vi "roverView.vi"() -> ()   [LabVIEW 2020]
uses:
  globalVariables.vi
panel:
  in  "Simulation stop":bool
  out "Back right wheel":dbl(graph)
  out "Back left wheel":dbl(graph)
  out "Front right wheel":dbl(graph)
  out "Front left wheel":dbl(graph)
  out "Velocity of the rover's left-side wheels":dbl(graph)
  out "Rover wheel velocity on the right side":string
  out "Scientific notation":dbl
  out "Scientific notation":dbl
  out "Rover wheel velocity on the left side":string
  out "Velocity of the rover's right-side wheels":dbl(graph)
  out "standard output 2":string
  out "ASCII Char 3":i16
  out "Character 2":string
  out "System user":string
  out "Simulation time":dbl
  out "Movement log":string
  out "Keys pressed log":string
  out "Key pressed":string
  out "Detected movement indicator":string
  out "ASCII Char 2":i16
  out "ASCII Char":i16
  out "Character":string
  out "standard output":string
  # "Rover control"
  # "Logs"
  # "Wheel movement charts"
  # "Movement data"
  # "Velocity charts"
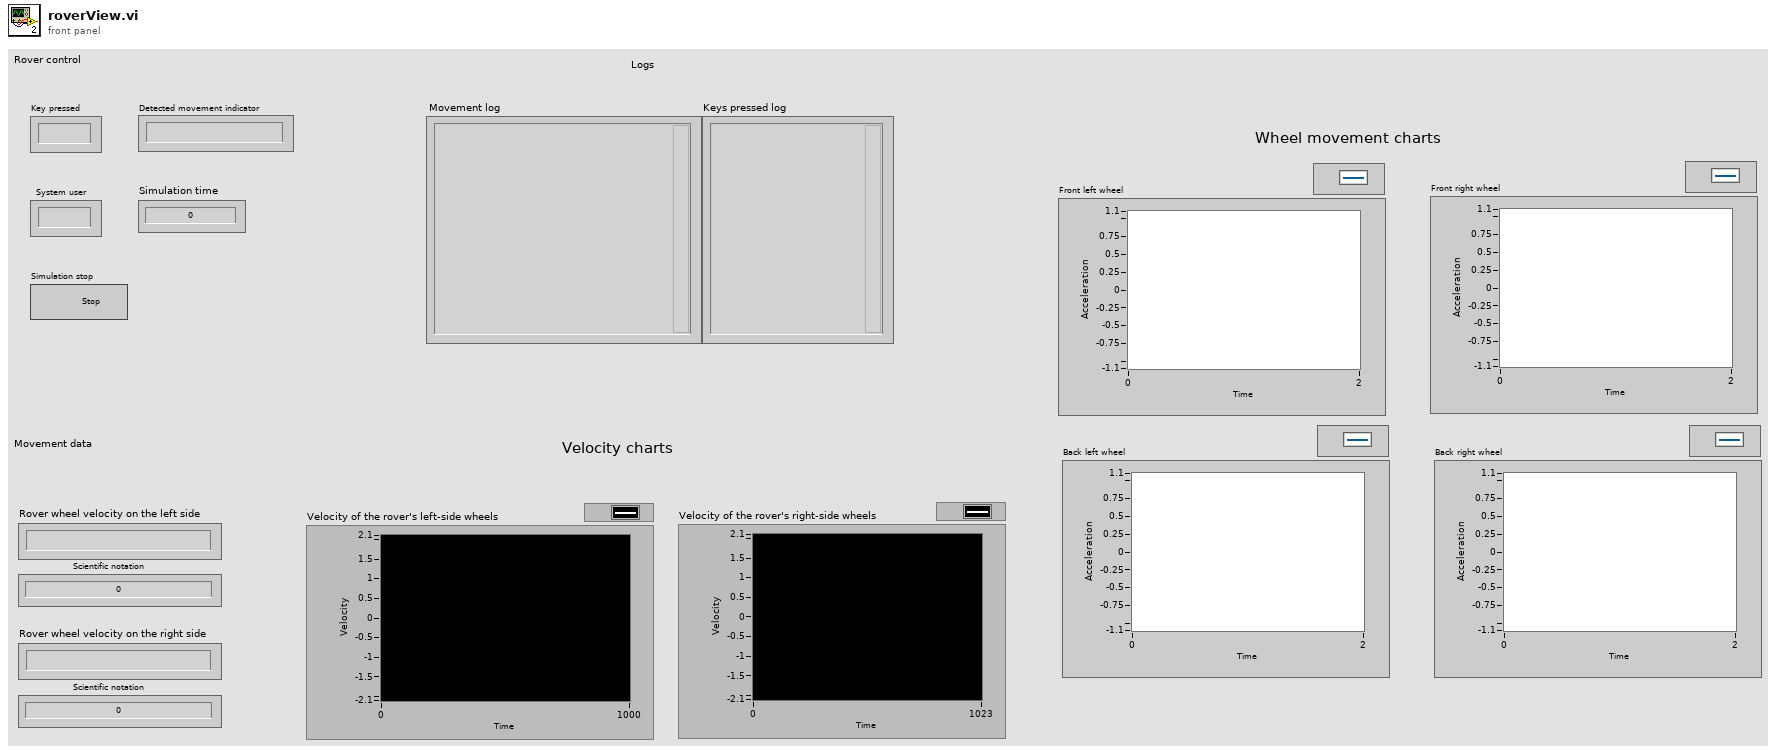
[diagram p1: front panel]
types:
  T1 = enum16{"Start", "Process 1", "Process 2", "Stop"}
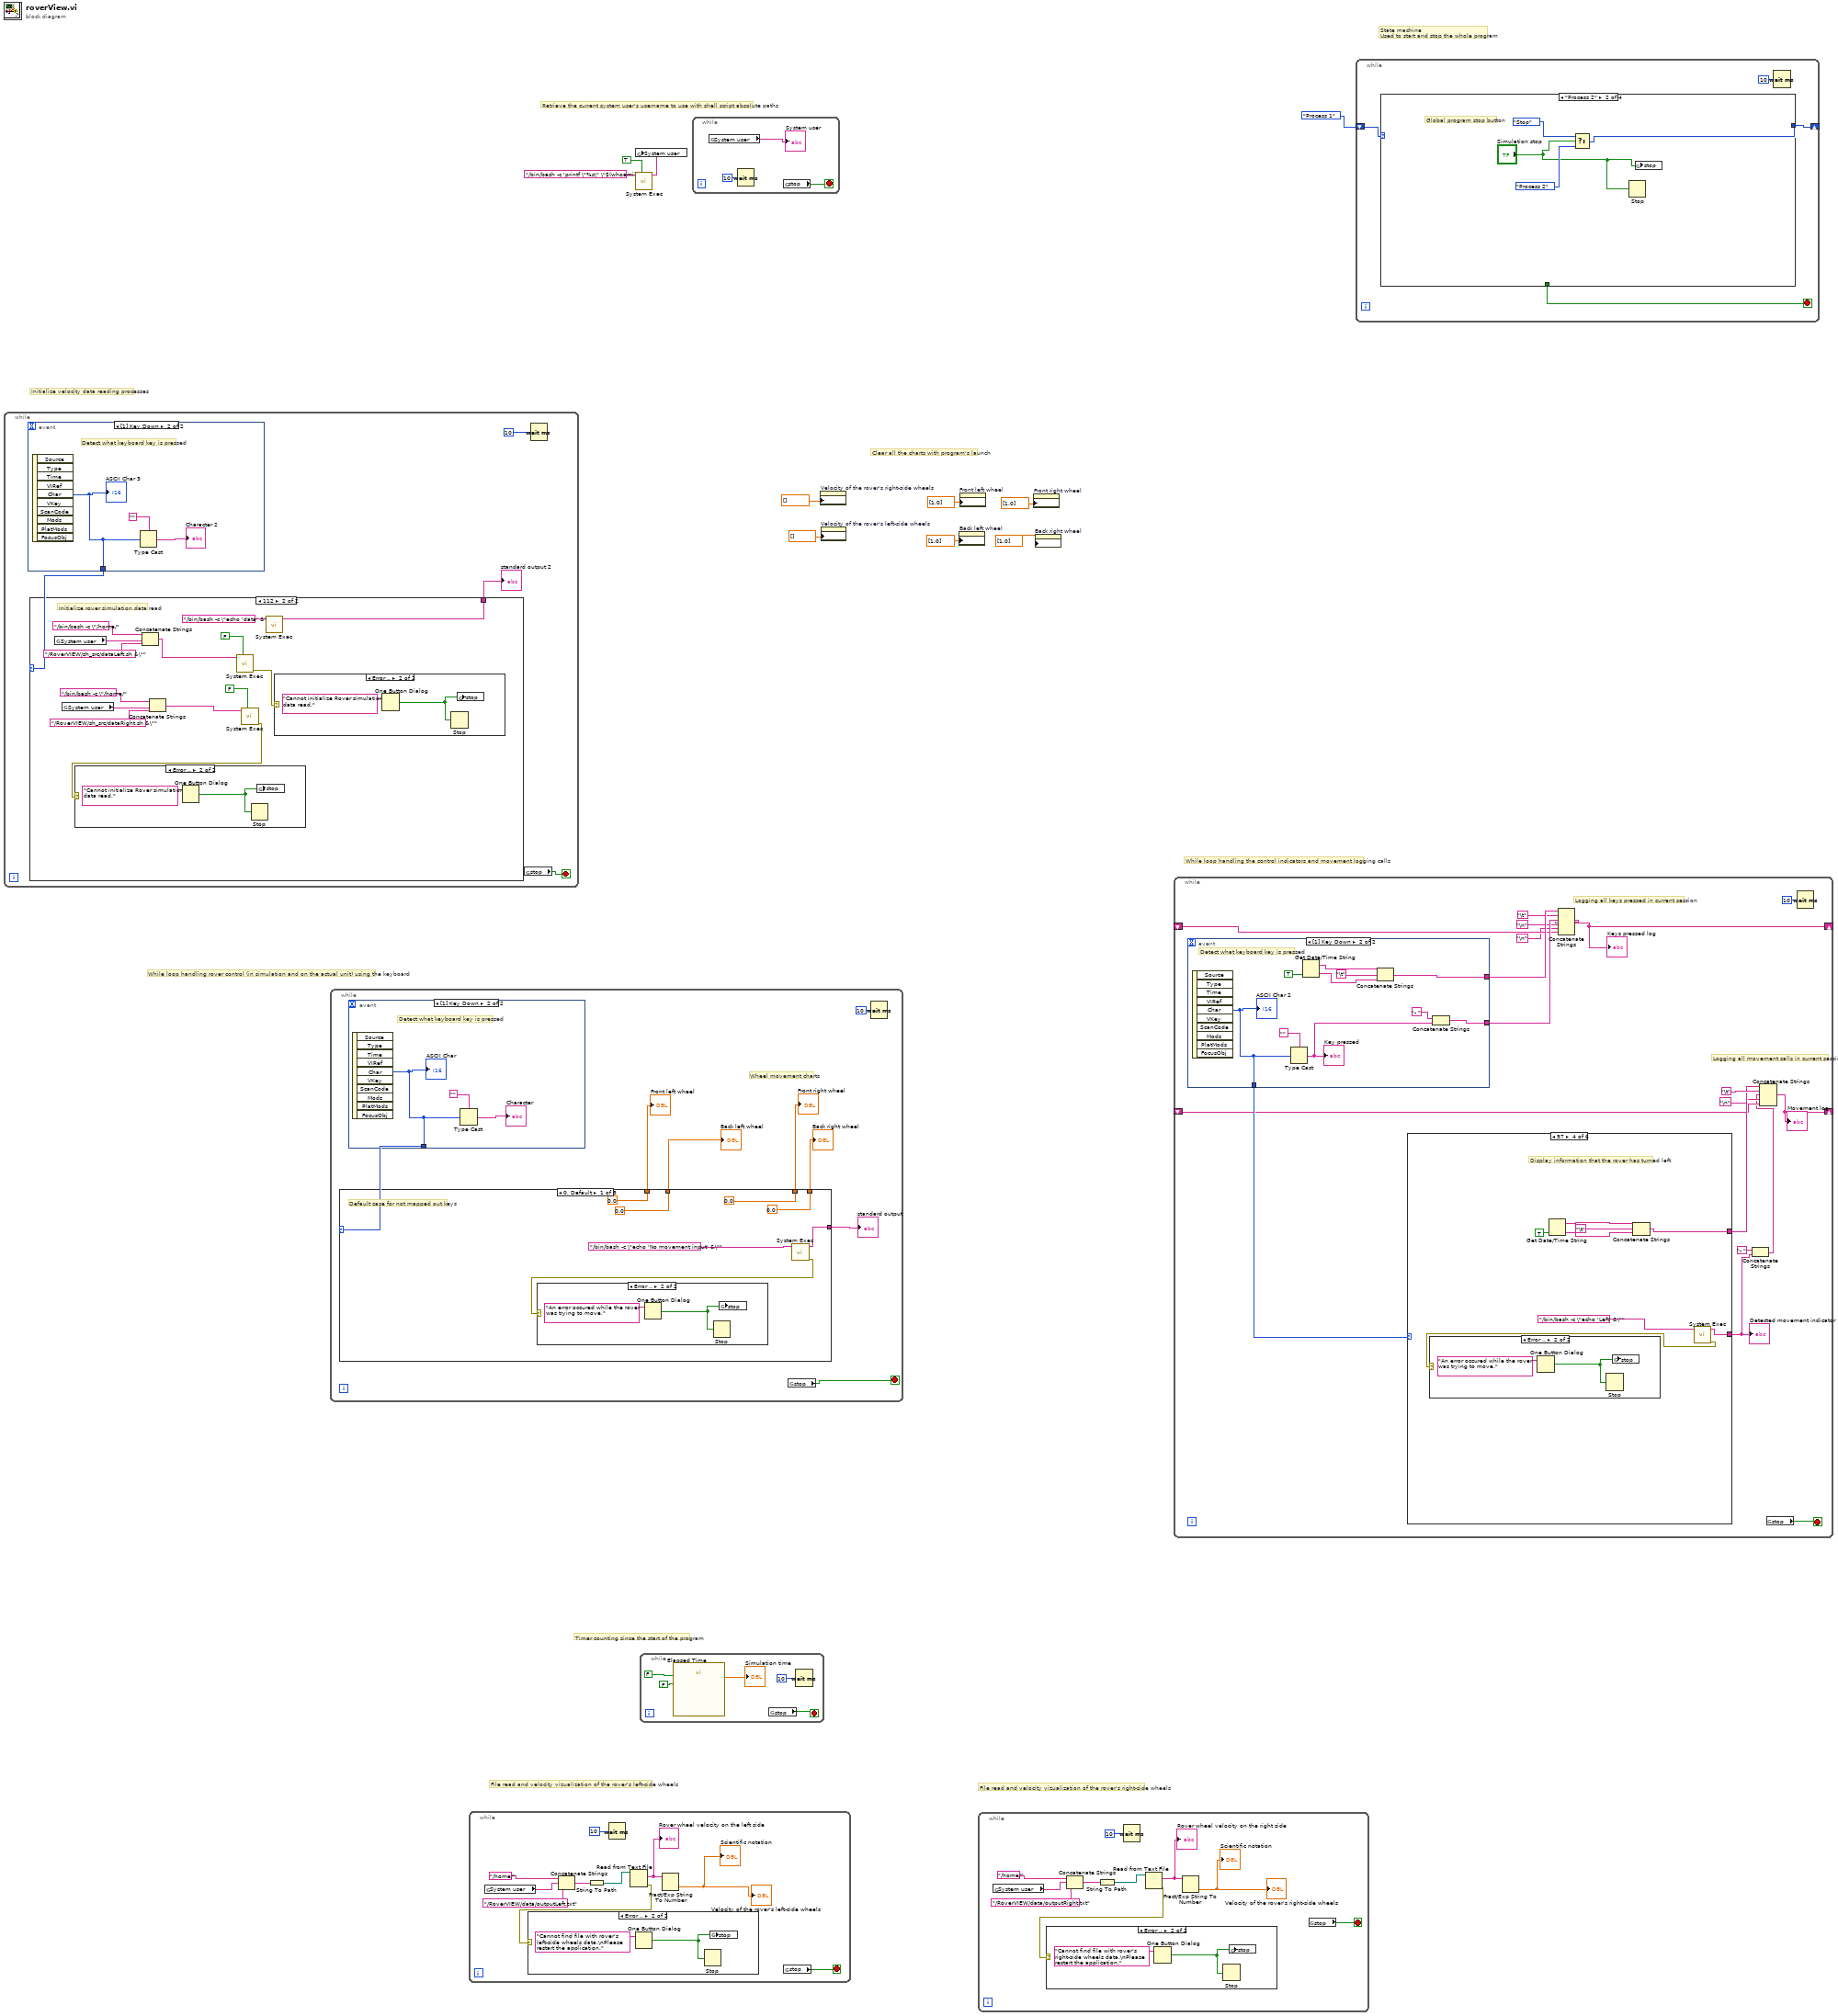
[diagram p0: block diagram]
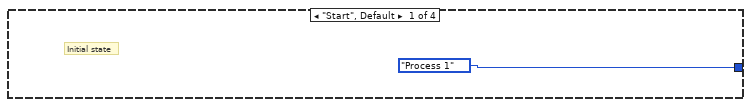
[diagram p2: hidden frame]
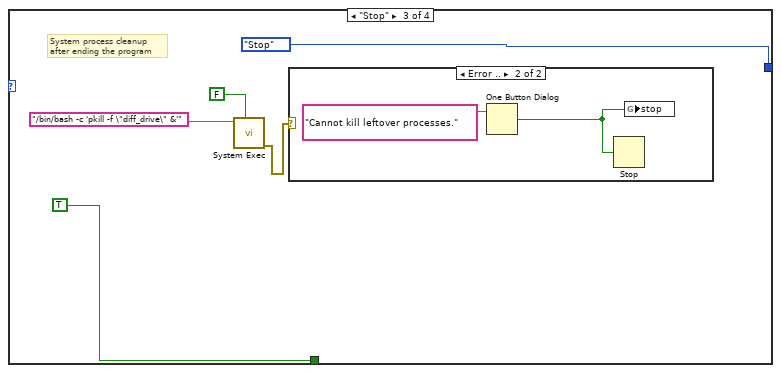
[diagram p3: hidden frame]
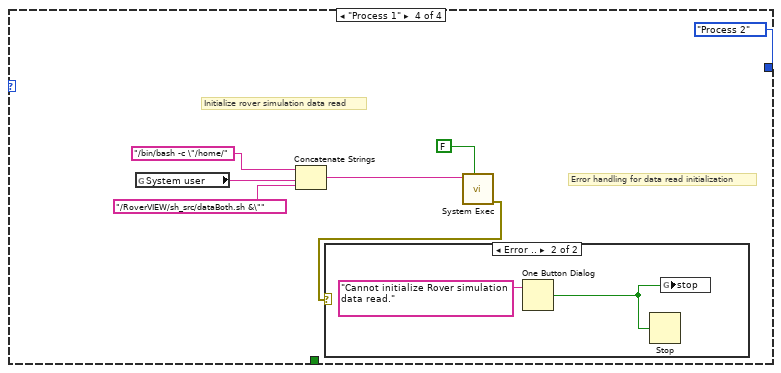
[diagram p5: hidden frame]
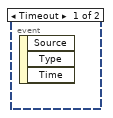
[diagram p7: hidden frame]
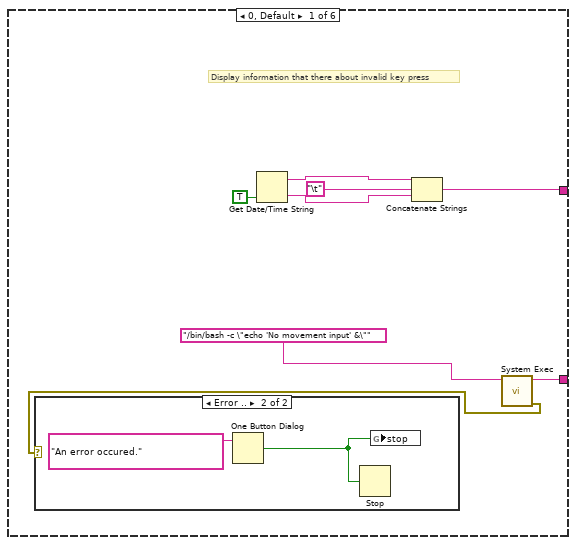
[diagram p13: hidden frame]
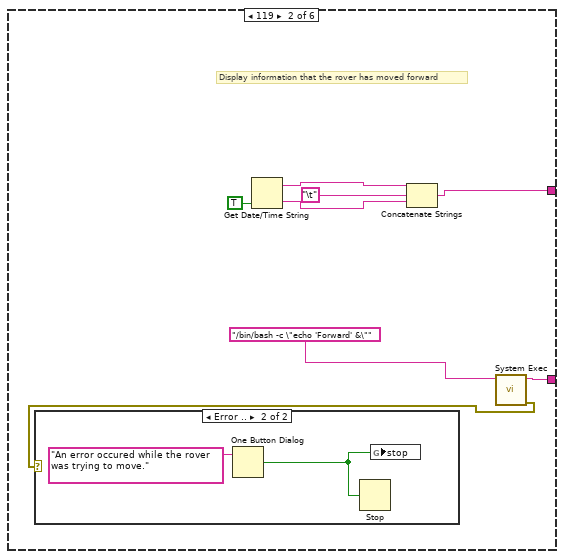
[diagram p15: hidden frame]
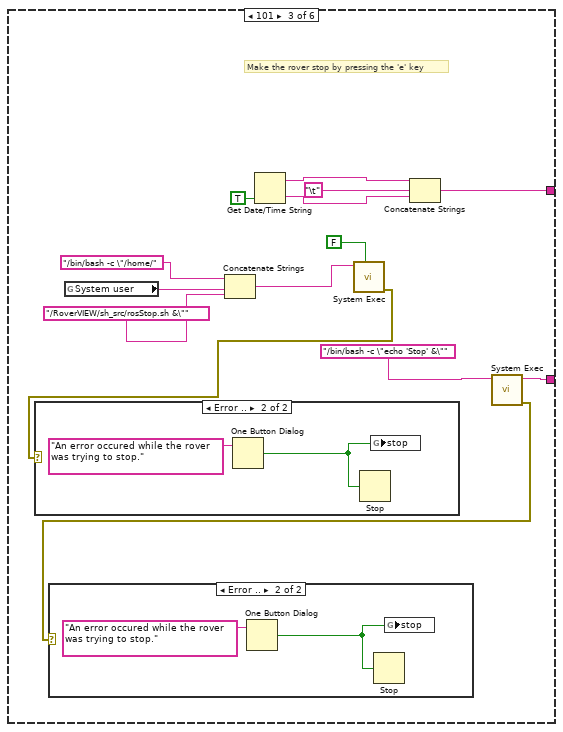
[diagram p17: hidden frame]
diagram:
  # "State machine\nUsed to start and stop the whole program"
  # "Clear all the charts with program's launch"
  # "Initialize velocity data reading processes"
  # "File read and velocity vizualization of the rover's right-side wheels"
  # "File read and velocity vizualization of the rover's left-side wheels"
  # "Timer counting since the start of the program"
  # "Retrieve the current system user's username to use with shell script absolute paths"
  # "While loop handling the control indicators and movement logging calls"
  # "While loop handling rover control (in simulation and on the actual unit) using the keyboard"
  n1 = while {
    stop <- w11 stop-if-true
    n2 = event shown="[1] Key Down" {
      selector: _ -> [_ _]
      dyn-events: _ -> [_ _]
      timeout: _ -> [_ _]
      tunnel: [_ w15] -> w14
      event Timeout {
        n3 = event-data() -> ()  [unwired: 1 in, 3 out]
      }
      event Key Down {
        # "Detect what keyboard key is pressed"
        n4 = event-data() -> ("Char"=w15:i16)  [unwired: 1 in, 9 out]
        "ASCII Char 3" <- w15
        n5 = Type Cast(type="", x=w15) -> (*(type *) &x=→"Character 2":string)
      }
    }
    n6 = case shown="112" w14 {
      tunnel: [_ w28] -> w13
      frame 0, Default {
        # "Initial state"
      }
      frame 112 {
        # "Initialize rover simulation data read"
        n7 = global read "globalVariables.vi" "System user"() -> (w22:string)
        n8 = global read "globalVariables.vi" "System user"() -> (w26:string)
        n9 = Concatenate Strings("/bin/bash -c \"/home/", w22, "/RoverVIEW/sh_src/dataLeft.sh &\"") -> (w20:string)
        n10 = Concatenate Strings("/bin/bash -c \"/home/", w26, "/RoverVIEW/sh_src/dataRight.sh &\"") -> (w24:string)
        n11 = call <vilib>:"System Exec.vi"("wait until completion? (T)"=FALSE, "command line"=w20) -> ("error out"=w18:errorcluster)  [unwired: 6 in, 3 out]
        n12 = call <vilib>:"System Exec.vi"("wait until completion? (T)"=FALSE, "command line"=w24) -> ("error out"=w19:errorcluster)  [unwired: 6 in, 3 out]
        n13 = case shown="Error .." w19 {
          frame No Error {
          }
          frame Error {
            n14 = One Button Dialog(message="Cannot initialize Rover simulation data read.") -> (true=w34:bool)  [unwired: 1 in]
            n15 = Stop(stop? (T)=w34) -> ()
            n16 = global write "globalVariables.vi" "stop"(w34) -> ()
          }
        }
        n17 = call <vilib>:"System Exec.vi"("command line"="/bin/bash -c \"echo 'data' &\"") -> ("standard output"=w28:string)  [unwired: 7 in, 3 out]
        n18 = case shown="Error .." w18 {
          frame No Error {
          }
          frame Error {
            n19 = One Button Dialog(message="Cannot initialize Rover simulation data read.") -> (true=w32:bool)  [unwired: 1 in]
            n20 = Stop(stop? (T)=w32) -> ()
            n21 = global write "globalVariables.vi" "stop"(w32) -> ()
          }
        }
      }
    }
    "standard output 2" <- w13
    n22 = global read "globalVariables.vi" "stop"() -> (w11:bool)
    n23 = Wait (ms)(milliseconds to wait=u32 10) -> ()  [unwired: 1 out]
  }
  n24 = while {
    stop <- w36 stop-if-true
    # "Wheel movement charts"
    n25 = event shown="[1] Key Down" {
      selector: _ -> [_ _]
      dyn-events: _ -> [_ _]
      timeout: _ -> [_ _]
      tunnel: [_ w105] -> w43
      event Timeout {
        n26 = event-data() -> ()  [unwired: 1 in, 3 out]
      }
      event Key Down {
        # "Detect what keyboard key is pressed"
        n27 = event-data() -> ("Char"=w105:i16)  [unwired: 1 in, 9 out]
        "ASCII Char" <- w105
        n28 = Type Cast(type="", x=w105) -> (*(type *) &x=→"Character":string)
      }
    }
    n29 = case shown="0, Default" w43 {
      tunnel: [w49 w63 w76 w89 w102] -> w42
      tunnel: [0.0 1.0 0.0 -1.0 1.0] -> w37
      tunnel: [0.0 1.0 0.0 -1.0 1.0] -> w40
      tunnel: [0.0 1.0 1.0 -1.0 0.0] -> w39
      tunnel: [0.0 1.0 1.0 -1.0 0.0] -> w38
      frame 0, Default {
        # "Default case for not mapped out keys"
        n30 = call <vilib>:"System Exec.vi"("command line"="/bin/bash -c \"echo 'No movement input' &\"") -> ("error out"=w44:errorcluster, "standard output"=w49:string)  [unwired: 7 in, 2 out]
        n31 = case shown="Error .." w44 {
          frame No Error {
          }
          frame Error {
            n32 = One Button Dialog(message="An error occured while the rover was trying to move.") -> (true=w51:bool)  [unwired: 1 in]
            n33 = Stop(stop? (T)=w51) -> ()
            n34 = global write "globalVariables.vi" "stop"(w51) -> ()
          }
        }
      }
      frame 119 {
        # "Make the rover move forward by pressing the 'w' key"
        n35 = global read "globalVariables.vi" "System user"() -> (w60:string)
        n36 = Concatenate Strings("/bin/bash -c \"/home/", w60, "/RoverVIEW/sh_src/rosForward.sh &\"") -> (w58:string)
        n37 = call <vilib>:"System Exec.vi"("wait until completion? (T)"=FALSE, "command line"=w58) -> ("error out"=w53:errorcluster, "standard output"=w63:string)  [unwired: 6 in, 2 out]
        n38 = case shown="Error .." w53 {
          frame No Error {
          }
          frame Error {
            n39 = One Button Dialog(message="An error occured while the rover was trying to move.") -> (true=w64:bool)  [unwired: 1 in]
            n40 = Stop(stop? (T)=w64) -> ()
            n41 = global write "globalVariables.vi" "stop"(w64) -> ()
          }
        }
      }
      frame 97 {
        # "Make the rover move left by pressing the 'a' key"
        n42 = global read "globalVariables.vi" "System user"() -> (w73:string)
        n43 = Concatenate Strings("/bin/bash -c \"/home/", w73, "/RoverVIEW/sh_src/rosLeft.sh &\"") -> (w71:string)
        n44 = call <vilib>:"System Exec.vi"("wait until completion? (T)"=FALSE, "command line"=w71) -> ("error out"=w66:errorcluster, "standard output"=w76:string)  [unwired: 6 in, 2 out]
        n45 = case shown="Error .." w66 {
          frame No Error {
          }
          frame Error {
            n46 = One Button Dialog(message="An error occured while the rover was trying to move.") -> (true=w77:bool)  [unwired: 1 in]
            n47 = Stop(stop? (T)=w77) -> ()
            n48 = global write "globalVariables.vi" "stop"(w77) -> ()
          }
        }
      }
      frame 115 {
        # "Make the rover move backwards by pressing the 's' key"
        n49 = global read "globalVariables.vi" "System user"() -> (w86:string)
        n50 = Concatenate Strings("/bin/bash -c \"/home/", w86, "/RoverVIEW/sh_src/rosBackwards.sh &\"") -> (w84:string)
        n51 = call <vilib>:"System Exec.vi"("wait until completion? (T)"=FALSE, "command line"=w84) -> ("error out"=w79:errorcluster, "standard output"=w89:string)  [unwired: 6 in, 2 out]
        n52 = case shown="Error .." w79 {
          frame No Error {
          }
          frame Error {
            n53 = One Button Dialog(message="An error occured while the rover was trying to move.") -> (true=w90:bool)  [unwired: 1 in]
            n54 = Stop(stop? (T)=w90) -> ()
            n55 = global write "globalVariables.vi" "stop"(w90) -> ()
          }
        }
      }
      frame 100 {
        # "Make the rover move right by pressing the 'd' key"
        n56 = global read "globalVariables.vi" "System user"() -> (w99:string)
        n57 = Concatenate Strings("/bin/bash -c \"/home/", w99, "/RoverVIEW/sh_src/rosRight.sh &\"") -> (w97:string)
        n58 = call <vilib>:"System Exec.vi"("wait until completion? (T)"=FALSE, "command line"=w97) -> ("error out"=w92:errorcluster, "standard output"=w102:string)  [unwired: 6 in, 2 out]
        n59 = case shown="Error .." w92 {
          frame No Error {
          }
          frame Error {
            n60 = One Button Dialog(message="An error occured while the rover was trying to move.") -> (true=w103:bool)  [unwired: 1 in]
            n61 = Stop(stop? (T)=w103) -> ()
            n62 = global write "globalVariables.vi" "stop"(w103) -> ()
          }
        }
      }
    }
    "standard output" <- w42
    "Front left wheel" <- w37
    "Front right wheel" <- w39
    "Back left wheel" <- w40
    "Back right wheel" <- w38
    n63 = global read "globalVariables.vi" "stop"() -> (w36:bool)
    n64 = Wait (ms)(milliseconds to wait=u32 10) -> ()  [unwired: 1 out]
  }
  n65 = while {
    stop <- w109 stop-if-true
    n66 = global read "globalVariables.vi" "System user"() -> (w114:string)
    n67 = Concatenate Strings("/home/", w114, "/RoverVIEW/data/outputLeft.txt") -> (w112:string)
    n68 = String To Path(string=w112) -> (path=w116:path)
    n69 = Wait (ms)(milliseconds to wait=u32 10) -> ()  [unwired: 1 out]
    n70 = Read from Text File(file (use dialog)=w116) -> (text=w111:string, error out=w108:errorcluster)  [unwired: 3 in, 2 out]
    "Rover wheel velocity on the left side" <- w111
    n71 = case shown="Error .." w108 {
      frame No Error {
      }
      frame Error {
        n72 = One Button Dialog(message="Cannot find file with rover's left-side wheels data.\nPlease restart the application.") -> (true=w118:bool)  [unwired: 1 in]
        n73 = Stop(stop? (T)=w118) -> ()
        n74 = global write "globalVariables.vi" "stop"(w118) -> ()
      }
    }
    n75 = Fract/Exp String To Number(string=w111) -> (number=→"Scientific notation" →"Velocity of the rover's left-side wheels":dbl)  [unwired: 3 in, 1 out]
    n76 = global read "globalVariables.vi" "stop"() -> (w109:bool)
  }
  n77 = call <vilib>:"System Exec.vi"("wait until completion? (T)"=TRUE, "command line"="/bin/bash -c 'printf \"%s\" \"$(whoami)\" &'") -> ("standard output"=w10:string)  [unwired: 6 in, 3 out]
  n78 = global write "globalVariables.vi" "System user"(w10) -> ()
  n79 = while {
    stop <- w121 stop-if-true
    n80 = call "Elapsed Time"("Reset"=FALSE, "Auto Reset"=FALSE) -> ("Elapsed Time (s)"=→"Simulation time":dbl)  [unwired: 10 in, 7 out]
    n81 = global read "globalVariables.vi" "stop"() -> (w121:bool)
    n82 = Wait (ms)(milliseconds to wait=u32 10) -> ()  [unwired: 1 out]
  }
  n83 = while {
    stop <- w125 stop-if-true
    n84 = global read "globalVariables.vi" "System user"() -> (→"System user":string)
    n85 = Wait (ms)(milliseconds to wait=u32 10) -> ()  [unwired: 1 out]
    n86 = global read "globalVariables.vi" "stop"() -> (w125:bool)
  }
  n87 = property on="Velocity of the rover's right-side wheels" class="WFChart (strict)"("History Data"=dbl[] []) -> ()  [unwired: 2 in, 2 out]
  n88 = property on="Velocity of the rover's left-side wheels" class="WFChart (strict)"("History Data"=dbl[] []) -> ()  [unwired: 2 in, 2 out]
  n89 = property on="Back left wheel" class="WFChart (strict)"("History Data"=dbl[] [1.0]) -> ()  [unwired: 2 in, 2 out]
  n90 = property on="Front left wheel" class="WFChart (strict)"("History Data"=dbl[] [1.0]) -> ()  [unwired: 2 in, 2 out]
  n91 = while {
    stop <- w129 stop-if-true
    n92 = global read "globalVariables.vi" "System user"() -> (w135:string)
    n93 = Concatenate Strings("/home/", w135, "/RoverVIEW/data/outputRight.txt") -> (w133:string)
    n94 = String To Path(string=w133) -> (path=w132:path)
    n95 = Wait (ms)(milliseconds to wait=u32 10) -> ()  [unwired: 1 out]
    n96 = Read from Text File(file (use dialog)=w132) -> (text=w130:string, error out=w128:errorcluster)  [unwired: 3 in, 2 out]
    "Rover wheel velocity on the right side" <- w130
    n97 = case shown="Error .." w128 {
      frame No Error {
      }
      frame Error {
        n98 = One Button Dialog(message="Cannot find file with rover's right-side wheels data.\nPlease restart the application.") -> (true=w138:bool)  [unwired: 1 in]
        n99 = Stop(stop? (T)=w138) -> ()
        n100 = global write "globalVariables.vi" "stop"(w138) -> ()
      }
    }
    n101 = Fract/Exp String To Number(string=w130) -> (number=→"Velocity of the rover's right-side wheels" →"Scientific notation":dbl)  [unwired: 3 in, 1 out]
    n102 = global read "globalVariables.vi" "stop"() -> (w129:bool)
  }
  n103 = property on="Front right wheel" class="WFChart (strict)"("History Data"=dbl[] [1.0]) -> ()  [unwired: 2 in, 2 out]
  n104 = property on="Back right wheel" class="WFChart (strict)"("History Data"=dbl[] [1.0]) -> ()  [unwired: 2 in, 2 out]
  n105 = while {
    shift-right: [w151] -> _
    shift-left: _ -> [w142]
    shift-right: [w150] -> _
    shift-left: _ -> [w146]
    stop <- w140 stop-if-true
    # "Logging all movement calls in current session"
    # "Logging all keys pressed in current session"
    n106 = event shown="[1] Key Down" {
      selector: _ -> [_ _]
      dyn-events: _ -> [_ _]
      timeout: _ -> [_ _]
      tunnel: [_ w234] -> w157
      tunnel: [_ w230] -> w155
      tunnel: [_ w226] -> w154
      event Timeout {
        n107 = event-data() -> ()  [unwired: 1 in, 3 out]
      }
      event Key Down {
        # "Detect what keyboard key is pressed"
        n108 = event-data() -> ("Char"=w234:i16)  [unwired: 1 in, 9 out]
        "ASCII Char 2" <- w234
        n109 = Type Cast(type="", x=w234) -> (*(type *) &x=w227:string)
        "Key pressed" <- w227
        n110 = Get Date/Time String(want seconds? (F)=TRUE) -> (date string=w232:string, time string=w231:string)  [unwired: 2 in]
        n111 = Concatenate Strings(w232, "\t", w231) -> (w230:string)
        n112 = Concatenate Strings("- " ("string"), w227) -> (w226:string)
      }
    }
    n113 = case shown="97" w157 {
      tunnel: [w164 w174 w190 w202 w212 w222] -> w143
      tunnel: [w159 w169 w184 w197 w207 w217] -> w148
      frame 0, Default {
        # "Display information that there about invalid key press"
        n114 = Get Date/Time String(want seconds? (F)=TRUE) -> (date string=w160:string, time string=w161:string)  [unwired: 2 in]
        n115 = Concatenate Strings(w160, "\t", w161) -> (w159:string)
        n116 = call <vilib>:"System Exec.vi"("command line"="/bin/bash -c \"echo 'No movement input' &\"") -> ("error out"=w158:errorcluster, "standard output"=w164:string)  [unwired: 7 in, 2 out]
        n117 = case shown="Error .." w158 {
          frame No Error {
          }
          frame Error {
            n118 = One Button Dialog(message="An error occured.") -> (true=w166:bool)  [unwired: 1 in]
            n119 = Stop(stop? (T)=w166) -> ()
            n120 = global write "globalVariables.vi" "stop"(w166) -> ()
          }
        }
      }
      frame 119 {
        # "Display information that the rover has moved forward"
        n121 = Get Date/Time String(want seconds? (F)=TRUE) -> (date string=w170:string, time string=w171:string)  [unwired: 2 in]
        n122 = Concatenate Strings(w170, "\t", w171) -> (w169:string)
        n123 = call <vilib>:"System Exec.vi"("command line"="/bin/bash -c \"echo 'Forward' &\"") -> ("error out"=w168:errorcluster, "standard output"=w174:string)  [unwired: 7 in, 2 out]
        n124 = case shown="Error .." w168 {
          frame No Error {
          }
          frame Error {
            n125 = One Button Dialog(message="An error occured while the rover was trying to move.") -> (true=w176:bool)  [unwired: 1 in]
            n126 = Stop(stop? (T)=w176) -> ()
            n127 = global write "globalVariables.vi" "stop"(w176) -> ()
          }
        }
      }
      frame 101 {
        # "Make the rover stop by pressing the 'e' key"
        n128 = global read "globalVariables.vi" "System user"() -> (w182:string)
        n129 = Concatenate Strings("/bin/bash -c \"/home/", w182, "/RoverVIEW/sh_src/rosStop.sh &\"") -> (w180:string)
        n130 = Get Date/Time String(want seconds? (F)=TRUE) -> (date string=w185:string, time string=w186:string)  [unwired: 2 in]
        n131 = call <vilib>:"System Exec.vi"("wait until completion? (T)"=FALSE, "command line"=w180) -> ("error out"=w179:errorcluster)  [unwired: 6 in, 3 out]
        n132 = case shown="Error .." w179 {
          frame No Error {
          }
          frame Error {
            n133 = One Button Dialog(message="An error occured while the rover was trying to stop.") -> (true=w194:bool)  [unwired: 1 in]
            n134 = Stop(stop? (T)=w194) -> ()
            n135 = global write "globalVariables.vi" "stop"(w194) -> ()
          }
        }
        n136 = Concatenate Strings(w185, "\t", w186) -> (w184:string)
        n137 = call <vilib>:"System Exec.vi"("command line"="/bin/bash -c \"echo 'Stop' &\"") -> ("error out"=w178:errorcluster, "standard output"=w190:string)  [unwired: 7 in, 2 out]
        n138 = case shown="Error .." w178 {
          frame No Error {
          }
          frame Error {
            n139 = One Button Dialog(message="An error occured while the rover was trying to stop.") -> (true=w192:bool)  [unwired: 1 in]
            n140 = Stop(stop? (T)=w192) -> ()
            n141 = global write "globalVariables.vi" "stop"(w192) -> ()
          }
        }
      }
      frame 97 {
        # "Display information that the rover has turned left"
        n142 = Get Date/Time String(want seconds? (F)=TRUE) -> (date string=w198:string, time string=w199:string)  [unwired: 2 in]
        n143 = Concatenate Strings(w198, "\t", w199) -> (w197:string)
        n144 = call <vilib>:"System Exec.vi"("command line"="/bin/bash -c \"echo 'Left' &\"") -> ("error out"=w196:errorcluster, "standard output"=w202:string)  [unwired: 7 in, 2 out]
        n145 = case shown="Error .." w196 {
          frame No Error {
          }
          frame Error {
            n146 = One Button Dialog(message="An error occured while the rover was trying to move.") -> (true=w204:bool)  [unwired: 1 in]
            n147 = Stop(stop? (T)=w204) -> ()
            n148 = global write "globalVariables.vi" "stop"(w204) -> ()
          }
        }
      }
      frame 115 {
        # "Display information that the rover has moved backwards"
        n149 = Get Date/Time String(want seconds? (F)=TRUE) -> (date string=w208:string, time string=w209:string)  [unwired: 2 in]
        n150 = Concatenate Strings(w208, "\t", w209) -> (w207:string)
        n151 = call <vilib>:"System Exec.vi"("command line"="/bin/bash -c \"echo 'Backwards' &\"") -> ("error out"=w206:errorcluster, "standard output"=w212:string)  [unwired: 7 in, 2 out]
        n152 = case shown="Error .." w206 {
          frame No Error {
          }
          frame Error {
            n153 = One Button Dialog(message="An error occured while the rover was trying to move.") -> (true=w214:bool)  [unwired: 1 in]
            n154 = Stop(stop? (T)=w214) -> ()
            n155 = global write "globalVariables.vi" "stop"(w214) -> ()
          }
        }
      }
      frame 100 {
        # "Display information that the rover has turned left"
        n156 = Get Date/Time String(want seconds? (F)=TRUE) -> (date string=w218:string, time string=w219:string)  [unwired: 2 in]
        n157 = Concatenate Strings(w218, "\t", w219) -> (w217:string)
        n158 = call <vilib>:"System Exec.vi"("command line"="/bin/bash -c \"echo 'Right' &\"") -> ("error out"=w216:errorcluster, "standard output"=w222:string)  [unwired: 7 in, 2 out]
        n159 = case shown="Error .." w216 {
          frame No Error {
          }
          frame Error {
            n160 = One Button Dialog(message="An error occured while the rover was trying to move.") -> (true=w224:bool)  [unwired: 1 in]
            n161 = Stop(stop? (T)=w224) -> ()
            n162 = global write "globalVariables.vi" "stop"(w224) -> ()
          }
        }
      }
    }
    "Detected movement indicator" <- w143
    n163 = Concatenate Strings(w155, "\t", w154, "\n", "\n", w142) -> (w151:string)
    "Keys pressed log" <- w151
    n164 = Concatenate Strings("- " ("string"), w143) -> (w145:string)
    n165 = Concatenate Strings(w148, "\t", w145, "\n", w146) -> (w150:string)
    "Movement log" <- w150
    n166 = global read "globalVariables.vi" "stop"() -> (w140:bool)
    n167 = Wait (ms)(milliseconds to wait=u32 10) -> ()  [unwired: 1 out]
  }
  n168 = while {
    shift-right: [w238] -> _
    shift-left: T1."Process 1" -> [w239]
    stop <- w236 stop-if-true
    n169 = case shown="\"Process 2\"" w239 {
      tunnel: [T1."Process 1" w243 T1."Stop" T1."Process 2"] -> w238
      tunnel: [_ _ TRUE _] -> w236
      frame "Start", Default {
        # "Initial state"
      }
      frame "Process 2" {
        # "Global program stop button"
        n170 = Select(t=T1."Stop", s="Simulation stop", f=T1."Process 2") -> (s? t:f=w243:T1)
        n171 = Stop(stop? (T)="Simulation stop") -> ()
        n172 = global write "globalVariables.vi" "stop"("Simulation stop") -> ()
      }
      frame "Stop" {
        # "System process cleanup\nafter ending the program"
        n173 = call <vilib>:"System Exec.vi"("wait until completion? (T)"=FALSE, "command line"="/bin/bash -c 'pkill -f \"diff_drive\" &'") -> ("error out"=w245:errorcluster)  [unwired: 6 in, 3 out]
        n174 = case shown="Error .." w245 {
          frame No Error {
          }
          frame Error {
            n175 = One Button Dialog(message="Cannot kill leftover processes.") -> (true=w250:bool)  [unwired: 1 in]
            n176 = Stop(stop? (T)=w250) -> ()
            n177 = global write "globalVariables.vi" "stop"(w250) -> ()
          }
        }
      }
      frame "Process 1" {
        # "Error handling for data read initialization"
        # "Initialize rover simulation data read"
        n178 = global read "globalVariables.vi" "System user"() -> (w256:string)
        n179 = Concatenate Strings("/bin/bash -c \"/home/", w256, "/RoverVIEW/sh_src/dataBoth.sh &\"") -> (w254:string)
        n180 = call <vilib>:"System Exec.vi"("wait until completion? (T)"=FALSE, "command line"=w254) -> ("error out"=w252:errorcluster)  [unwired: 6 in, 3 out]
        n181 = case shown="Error .." w252 {
          frame No Error {
          }
          frame Error {
            n182 = One Button Dialog(message="Cannot initialize Rover simulation data read.") -> (true=w259:bool)  [unwired: 1 in]
            n183 = Stop(stop? (T)=w259) -> ()
            n184 = global write "globalVariables.vi" "stop"(w259) -> ()
          }
        }
      }
    }
    n185 = Wait (ms)(milliseconds to wait=u32 10) -> ()  [unwired: 1 out]
  }
